vi "KE622x -- 2182 -A Set Params.vi"(0 "622x Resource In":refnum<visa-resource-name>, 1 "Check For SCPI Errors? (T)":bool=TRUE, 7 "2182 -A Params In":T1={"Auto Range?"=FALSE, "Man / Selected\n       Range"=enum."10mV", "Enable Digital\n       Filter?"=FALSE, "Filter Type"=enum."Movin", "Filter Count"=1, "      Filter\nWindow (%)"=0.01, "Enable Analog\n       Filter?"=FALSE, "NPLCs"=5} {"NPLCs" min=1 max=10; "Filter\nWindow (%)" min=0.01 max=10.0 step=0.01 format="%.2f"; "Filter Count" min=1 max=100}, 11 "error in (no error)":errorcluster) -> (4 "622x Resource Out (dupl)":refnum<visa-resource-name>, 15 "error out":errorcluster)   [LabVIEW 2013, in "Keithly user program.lvlib"]
uses:
  Keithly user program.lvlib
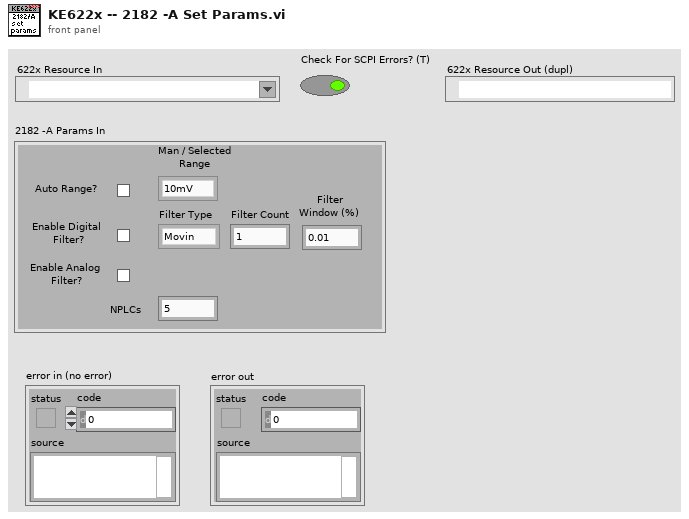
[diagram p1: front panel]
types:
  T1 = cluster{"Auto Range?":bool, "Man / Selected\n       Range":enum16{"10mV", "100mV", "1V", "10V", "100V"}, "Enable Digital\n       Filter?":bool, "Filter Type":enum16{"Movin", "Repeat"}, "Filter Count":u32, "      Filter\nWindow (%)":dbl, "Enable Analog\n       Filter?":bool, "NPLCs":u32}
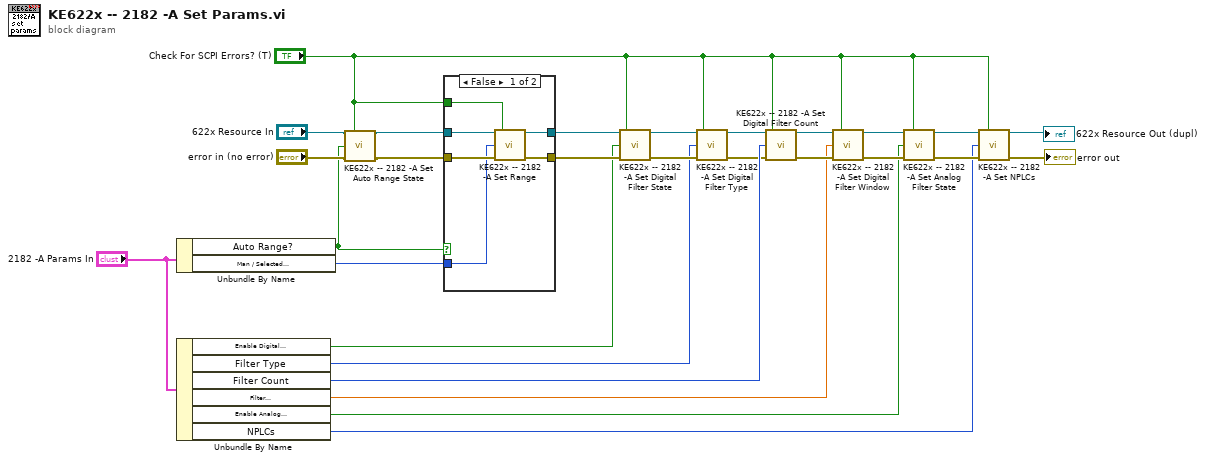
[diagram p0: block diagram]
diagram:
  n1 = Unbundle By Name("2182 -A Params In") -> ("Auto Range?"=w23:bool, "Man / Selected\n       Range"=w28:enum16{"10mV", "100mV", "1V", "10V", "100V"})
  n2 = Unbundle By Name("2182 -A Params In") -> ("Enable Digital\n       Filter?"=w20:bool, "Filter Type"=w17:enum16{"Movin", "Repeat"}, "Filter Count"=w15:u32, "Filter\nWindow (%)"=w11:dbl, "Enable Analog\n       Filter?"=w8:bool, "NPLCs"=w3:u32)
  n3 = call "KE622x -- 2182 -A Set Auto Range State.vi"("622x Resource In"="622x Resource In", "Check For SCPI Errors? (T)"="Check For SCPI Errors? (T)", "Enable Auto Range?"=w23, "error in (no error)"="error in (no error)") -> ("622x Resource Out (dupl)"=w27:refnum<visa-resource-name>, "error out"=w26:errorcluster)  [unwired: 10 in]
  n4 = case shown="False" w23 {
    tunnel: w27 -> [w34 w36]
    tunnel: w26 -> [w31 w35]
    tunnel: [w33 w36] -> w22
    tunnel: [w30 w35] -> w21
    tunnel: w28 -> [w29 _]
    tunnel: "Check For SCPI Errors? (T)" -> [w32 _]
    frame False {
      n5 = call "KE622x -- 2182 -A Set Range.vi"("622x Resource In"=w34, "Check For SCPI Errors? (T)"=w32, "2182/2182A Range"=w29, "error in (no error)"=w31) -> ("622x Resource Out (dupl)"=w33:refnum<visa-resource-name>, "error out"=w30:errorcluster)  [unwired: 10 in]
    }
    frame True {
    }
  }
  n6 = call "KE622x -- 2182 -A Set Digital Filter State.vi"("622x Resource In"=w22, "Check For SCPI Errors? (T)"="Check For SCPI Errors? (T)", "Enable Digital Filter?"=w20, "error in (no error)"=w21) -> ("622x Resource Out (dupl)"=w19:refnum<visa-resource-name>, "error out"=w18:errorcluster)  [unwired: 10 in]
  n7 = call "KE622x -- 2182 -A Set Digital Filter Type.vi"("622x Resource In"=w19, "Check For SCPI Errors? (T)"="Check For SCPI Errors? (T)", "Filter Type"=w17, "error in (no error)"=w18) -> ("622x Resource Out (dupl)"=w16:refnum<visa-resource-name>, "error out"=w14:errorcluster)  [unwired: 10 in]
  n8 = call "KE622x -- 2182 -A Set Digital Filter Count.vi"("622x Resource In"=w16, "Check For SCPI Errors? (T)"="Check For SCPI Errors? (T)", "Filter Count"=w15, "error in (no error)"=w14) -> ("622x Resource Out (dupl)"=w13:refnum<visa-resource-name>, "error out"=w12:errorcluster)  [unwired: 10 in]
  n9 = call "KE622x -- 2182 -A Set Digital Filter Window.vi"("622x Resource In"=w13, "Check For SCPI Errors? (T)"="Check For SCPI Errors? (T)", "Filter Window In (%)"=w11, "error in (no error)"=w12) -> ("622x Resource Out (dupl)"=w10:refnum<visa-resource-name>, "error out"=w9:errorcluster)  [unwired: 10 in]
  n10 = call "KE622x -- 2182 -A Set Analog Filter State.vi"("622x Resource In"=w10, "Check For SCPI Errors? (T)"="Check For SCPI Errors? (T)", "Enable Analog Filter?"=w8, "error in (no error)"=w9) -> ("622x Resource Out (dupl)"=w6:refnum<visa-resource-name>, "error out"=w5:errorcluster)  [unwired: 10 in]
  n11 = call "KE622x -- 2182 -A Set NPLCs.vi"("622x Resource In"=w6, "Check For SCPI Errors? (T)"="Check For SCPI Errors? (T)", "2182 -A NPLCs"=w3, "error in (no error)"=w5) -> ("622x Resource Out (dupl)"=→"622x Resource Out (dupl)":refnum<visa-resource-name>, "error out"=→"error out":errorcluster)  [unwired: 10 in]
